vi "WaitForData.vi"(8 "error in (no error)":errorcluster, 11 "Connection in":refnum<class "Connection.lvclass">) -> (0 "error out":errorcluster, 3 "Connection out":refnum<class "Connection.lvclass">)   [LabVIEW 2022 SP3, in "Connection.lvlib" / "Connection.lvclass"]
uses:
  Connection.lvclass
  <vilib>/ActorFramework/Actor/Actor.lvclass
  Connection Messages/Kill Msg/Kill Msg.lvclass
  Connection Messages/WaitForData Msg/WaitForData Msg.lvclass
  ReadData/ReadData.lvclass
  CallerMessage Messages/ConnectionDataRead Msg/ConnectionDataRead Msg.lvclass
  C:/Program Files (x86)/National Instruments/LabVIEW 2022/vi.lib/ActorFramework/Actor/Actor.lvclass
  TcpSocket/Source/TcpSocket/Connection/Connection.lvclass
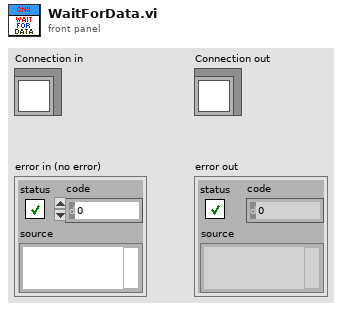
[diagram p1: front panel]
types:
  T1 = typedef "Connection.lvlib/Connection.lvclass/_State.ctl" = enum16{"WaitForInit", "Active", "Dying"}
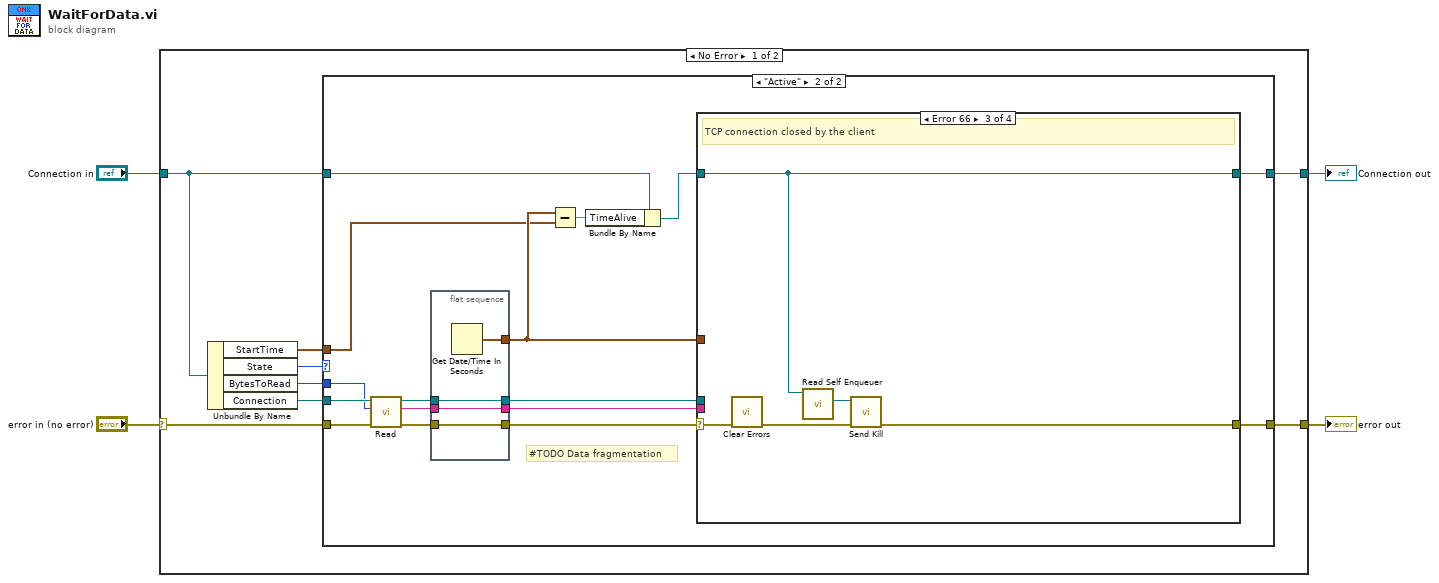
[diagram p0: block diagram]
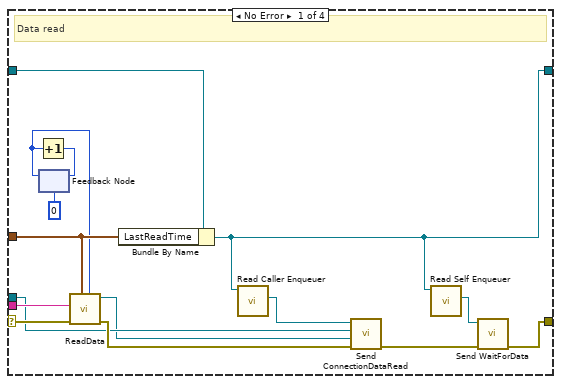
[diagram p3: hidden frame]
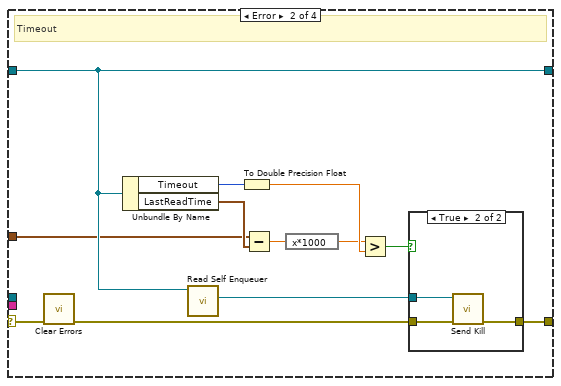
[diagram p4: hidden frame]
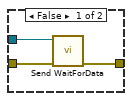
[diagram p5: hidden frame]
diagram:
  n1 = case shown="No Error" "error in (no error)" {
    selector: "error in (no error)" -> [w10 w76]
    tunnel: [w9 w76] -> w3
    tunnel: [w8 w75] -> w1
    tunnel: "Connection in" -> [w6 w75]
    frame No Error {
      n2 = Unbundle By Name(w6) -> ("StartTime"=w7:timestamp, "State"=w5:T1, "BytesToRead"=w11:i32, "Connection"=w12:refnum<class "Connection.lvclass">)
      n3 = case shown="\"Active\"" w5 {
        tunnel: w12 -> [_ w30]
        tunnel: w11 -> [_ w29]
        tunnel: w10 -> [w13 w28]
        tunnel: [w13 w27] -> w9
        tunnel: [w14 w22] -> w8
        tunnel: w7 -> [_ w18]
        tunnel: w6 -> [w14 w17]
        frame Default {
        }
        frame "Active" {
          # "#TODO Data fragmentation"
          n4 = call-dynamic "Read.vi"("error in (no error)"=w28, "BytesToRead"=w29, "Connection in"=w30) -> ("error out"=w25:errorcluster, "Data"=w23:string, "Connection out"=w15:refnum<class "Connection.lvclass">)  [unwired: 6 in]
          n5 = flat-sequence {
            tunnel: [w34] -> w26
            tunnel: w25 -> [w34]
            tunnel: [w33] -> w24
            tunnel: w23 -> [w33]
            tunnel: [w32] -> w21
            tunnel: [w31] -> w16
            tunnel: w15 -> [w31]
            frame #0 {
              n6 = Get Date/Time In Seconds() -> (seconds since 1Jan1904=w32:timestamp)
            }
          }
          n7 = Subtract(x=w21, y=w18) -> (x-y=w20:dbl)
          n8 = Bundle By Name(cluster=w17, "TimeAlive"=w20) -> (w19:refnum<class "Connection.lvclass">)
          n9 = case shown="Error 66" w26 {
            selector: w26 -> [w48 w56 w72 w74]
            tunnel: [w37 w57 w69 w74] -> w27
            tunnel: [w36 w54 w70 w73] -> w22
            tunnel: w19 -> [w49 w54 w70 w73]
            tunnel: w24 -> [w47 _ _ _]
            tunnel: w21 -> [w46 w52 _ _]
            tunnel: w16 -> [w40 _ _ _]
            frame No Error {
              # "Data read"
              n10 = feedback #1(u32 0) -> (w43:u32)
              n11 = Increment(x=w43) -> (x+1=w44:u32)
              n12 = feedback-in #1(w44) -> ()
              n13 = call "ReadData.vi"("ReadNumber"=w43, "TimeStamp"=w46, "error in (no error)"=w48, "Data"=w47) -> ("error out"=w42:errorcluster, "ReadData"=w39:refnum<class "ReadData.lvclass">)  [unwired: 6 in]
              n14 = Bundle By Name(cluster=w49, "LastReadTime"=w46) -> (w36:refnum<class "Connection.lvclass">)
              n15 = call <vilib>:"Read Caller Enqueuer.vi"("Actor"=w36) -> ("Caller Enqueuer"=w41:refnum<class "Message Enqueuer.lvclass">)  [unwired: 10 in]
              n16 = call "Send ConnectionDataRead.vi"("error in (no error)"=w42, "ReadData"=w39, "Connection"=w40, "Message Enqueuer"=w41) -> ("error out"=w38:errorcluster)  [unwired: 6 in, 1 out]
              n17 = call <vilib>:"Read Self Enqueuer.vi"("Actor"=w36) -> ("Self Enqueuer"=w35:refnum<class "Message Enqueuer.lvclass">)  [unwired: 10 in]
              n18 = call "Send WaitForData.vi"("error in (no error)"=w38, "Message Enqueuer"=w35) -> ("error out"=w37:errorcluster)  [unwired: 8 in, 1 out]
            }
            frame Error {
              # "Timeout"
              n19 = call <vilib>:"Clear Errors.vi"("error in (no error)"=w56) -> ("error out"=w51:errorcluster)  [unwired: 5 in, 1 out]
              n20 = Unbundle By Name(w54) -> ("Timeout"=w59:i32, "LastReadTime"=w61:timestamp)
              n21 = call <vilib>:"Read Self Enqueuer.vi"("Actor"=w54) -> ("Self Enqueuer"=w53:refnum<class "Message Enqueuer.lvclass">)  [unwired: 10 in]
              n22 = To Double Precision Float(number=w59) -> (double precision float=w58:dbl)
              n23 = Subtract(x=w52, y=w61) -> (x-y=w60:dbl)
              n24 = expression code="x*1000"(w60) -> (w50:dbl)
              n25 = Greater?(x=w50, y=w58) -> (0:w55:bool)
              n26 = case shown="True" w55 {
                tunnel: [w64 w66] -> w57
                tunnel: w51 -> [w63 w65]
                tunnel: w53 -> [w62 w67]
                frame False {
                  n27 = call "Send WaitForData.vi"("error in (no error)"=w63, "Message Enqueuer"=w62) -> ("error out"=w64:errorcluster)  [unwired: 8 in, 1 out]
                }
                frame True {
                  n28 = call "Send Kill.vi"("error in (no error)"=w65, "Message Enqueuer"=w67) -> ("error out"=w66:errorcluster)  [unwired: 8 in, 1 out]
                }
              }
            }
            frame Error {
              # "TCP connection closed by the client"
              n29 = call <vilib>:"Clear Errors.vi"("error in (no error)"=w72) -> ("error out"=w71:errorcluster)  [unwired: 5 in, 1 out]
              n30 = call <vilib>:"Read Self Enqueuer.vi"("Actor"=w70) -> ("Self Enqueuer"=w68:refnum<class "Message Enqueuer.lvclass">)  [unwired: 10 in]
              n31 = call "Send Kill.vi"("error in (no error)"=w71, "Message Enqueuer"=w68) -> ("error out"=w69:errorcluster)  [unwired: 8 in, 1 out]
            }
            frame Default {
              # "Error"
            }
          }
        }
      }
    }
    frame Error {
    }
  }
  "error out" <- w3
  "Connection out" <- w1
